vi "get_or_set_data_for_devices.vi"(7 "action":T1, 8 "error in (no error)":errorcluster, 10 "data for devices in":cluster{"data for channels":dbl[][]}[](array[cluster]), 11 "DAQmxWriteSignals in":refnum<class "SignalWriterMM140725DAQmx.lvclass">) -> (0 "error out":errorcluster, 2 "data for devices out":cluster{"data for channels":dbl[][]}[](array[cluster]), 3 "DAQmxWriteSignals out":refnum<class "SignalWriterMM140725DAQmx.lvclass">)   [LabVIEW 2010, in "SignalWriterMM140725DAQmx.lvclass"]
uses:
  SignalWriterMM140725DAQmx.lvclass
  common/enumerations/functional_global_action_enum.ctl
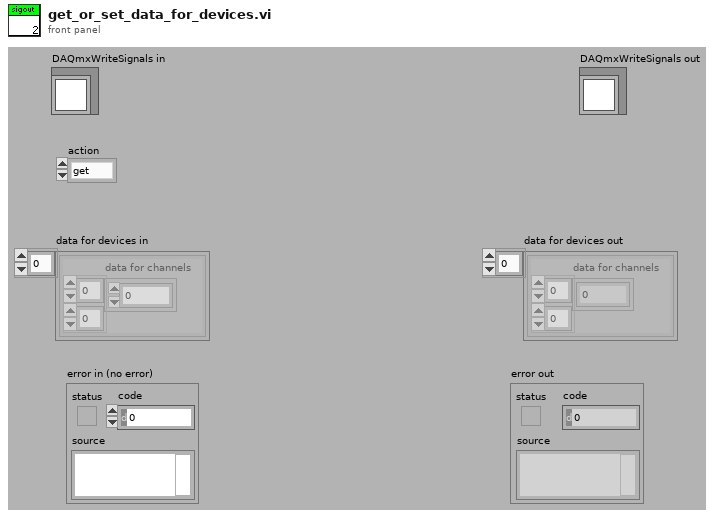
[diagram p1: front panel]
types:
  T1 = typedef "functional_global_action_enum.ctl" = enum16{"get", "set", "reset"}
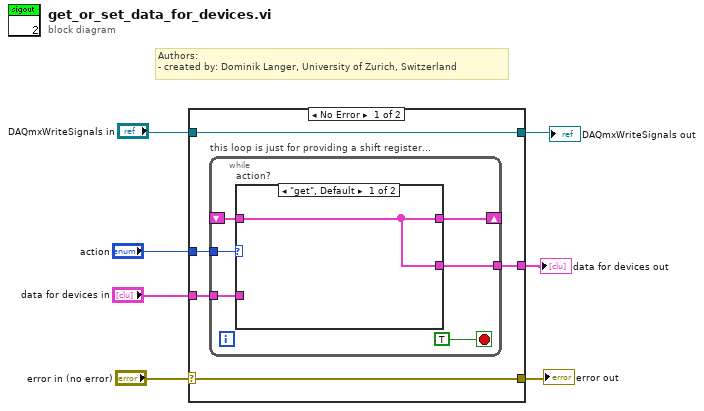
[diagram p0: block diagram]
diagram:
  # "Authors: \n- created by: Dominik Langer, University of Zurich, Switzerland"
  n1 = case shown="No Error" "error in (no error)" {
    selector: "error in (no error)" -> [w11 w22]
    tunnel: [w11 w22] -> w4
    tunnel: [w12 w21] -> w1
    tunnel: "DAQmxWriteSignals in" -> [w12 w21]
    tunnel: "action" -> [w10 _]
    tunnel: "data for devices in" -> [w9 _]
    tunnel: [w8 _] -> w5
    frame No Error {
      n2 = while "this loop is just for providing a shift register..." {
        tunnel: w10 -> [w18]
        tunnel: w9 -> [w17]
        tunnel: [w16] -> w8
        shift-right: [w14] -> _
        shift-left: _ -> [w13]
        stop <- TRUE stop-if-true
        n3 = case "action?" shown="\"get\", Default" w18 {
          tunnel: w17 -> [_ w20]
          tunnel: [w19 _] -> w16
          tunnel: [w19 w20] -> w14
          tunnel: w13 -> [w19 _]
          frame "get", Default {
          }
          frame "set" {
          }
        }
      }
    }
    frame Error {
    }
  }
  "error out" <- w4
  "data for devices out" <- w5
  "DAQmxWriteSignals out" <- w1
